vi "m100開機數統計.vi"() -> ()   [LabVIEW 2012]
uses:
  <vilib>/addons/database/Auxilliary.llb/DB Tools Cursor Type.ctl
  <vilib>/Utility/NIReport.llb/NI_report.lvclass
  <vilib>/addons/database/Connection.llb/DB Tools Open Connec (Path).vi
  <vilib>/addons/database/Connection.llb/Conn Execute.vi
  <vilib>/addons/database/Recordset.llb/Rec Fetch Recordset Data (R).vi
  <vilib>/addons/database/Recordset.llb/Rec Destroy - Connection.vi
  <vilib>/addons/database/Recordset.llb/Rec Fetch Integer Data (R).vi
  <vilib>/Utility/NIReport.llb/Append Text Table to Report (wrap).vi
  <vilib>/addons/database/_DB Variant To Data/Database Variant To Data.xnode
  <vilib>/addons/database/NI_Database_API.lvlib
  <vilib>/Utility/NIReport.llb/Excel/NI_Excel.lvclass
  <vilib>/addons/_office/NI_ReportGenerationToolkit.lvlib
panel:
  out "error out 2":errorcluster
  out "array":string[](array[string])
  out "data 3":i32
  out "data 2":string
  out "data":string
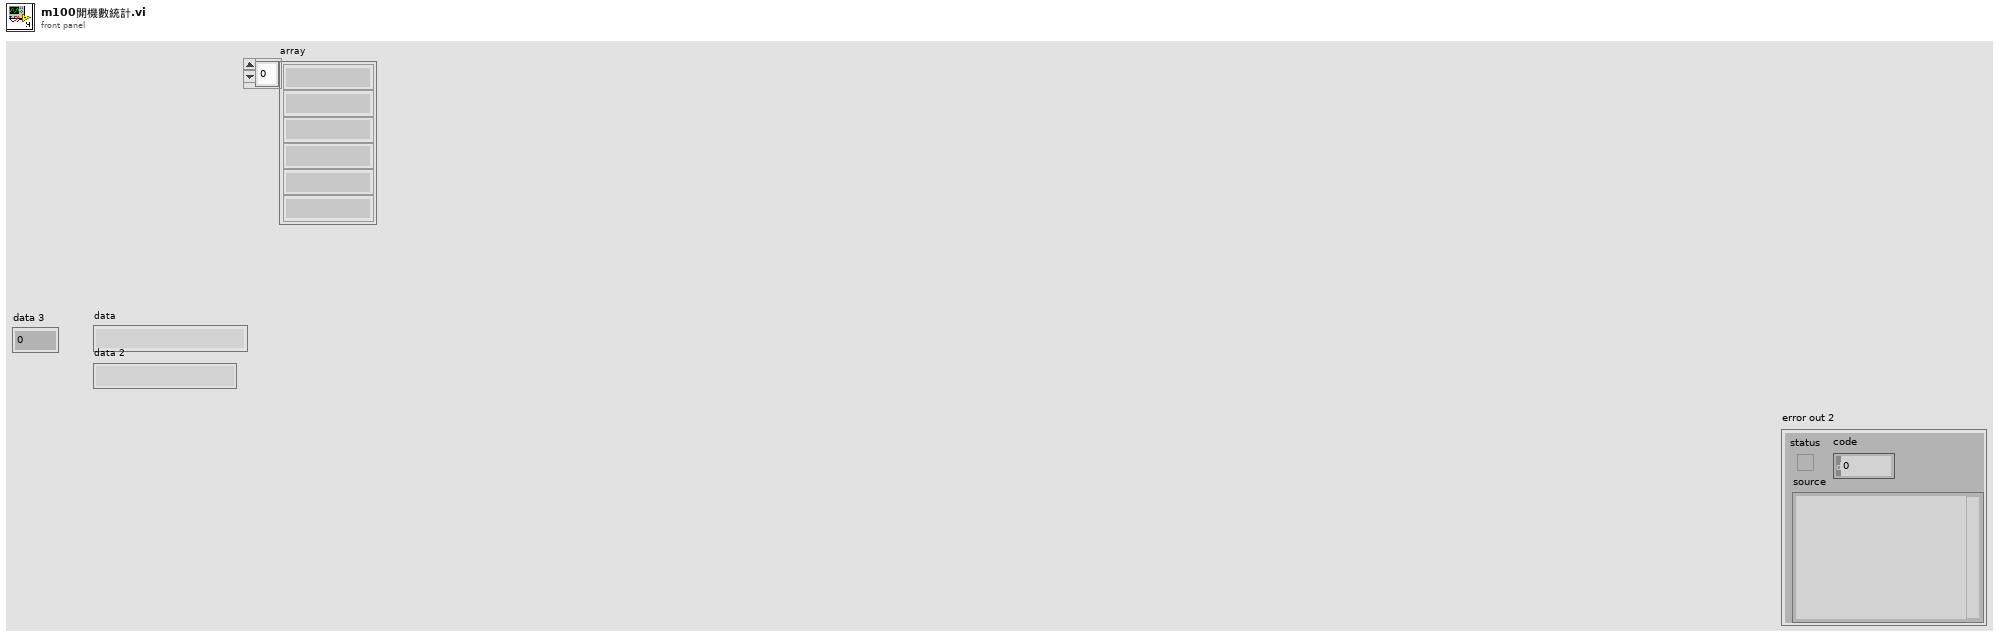
[diagram p1: front panel]
types:
  T1 = typedef "NI_Database_API.lvlib/DB Tools Cursor Type.ctl" = enum16{"forward-only", "keyset", "dynamic", "static"}
  T2 = typedef "NI_Database_API.lvlib/Conn ObjectReference.ctl" = refnum<k1>
  T3 = typedef "NI_Database_API.lvlib/Rec ObjectReference.ctl" = refnum<k1>
  T4 = enum16{"Standard Report", "HTML", "Word", "Excel"}
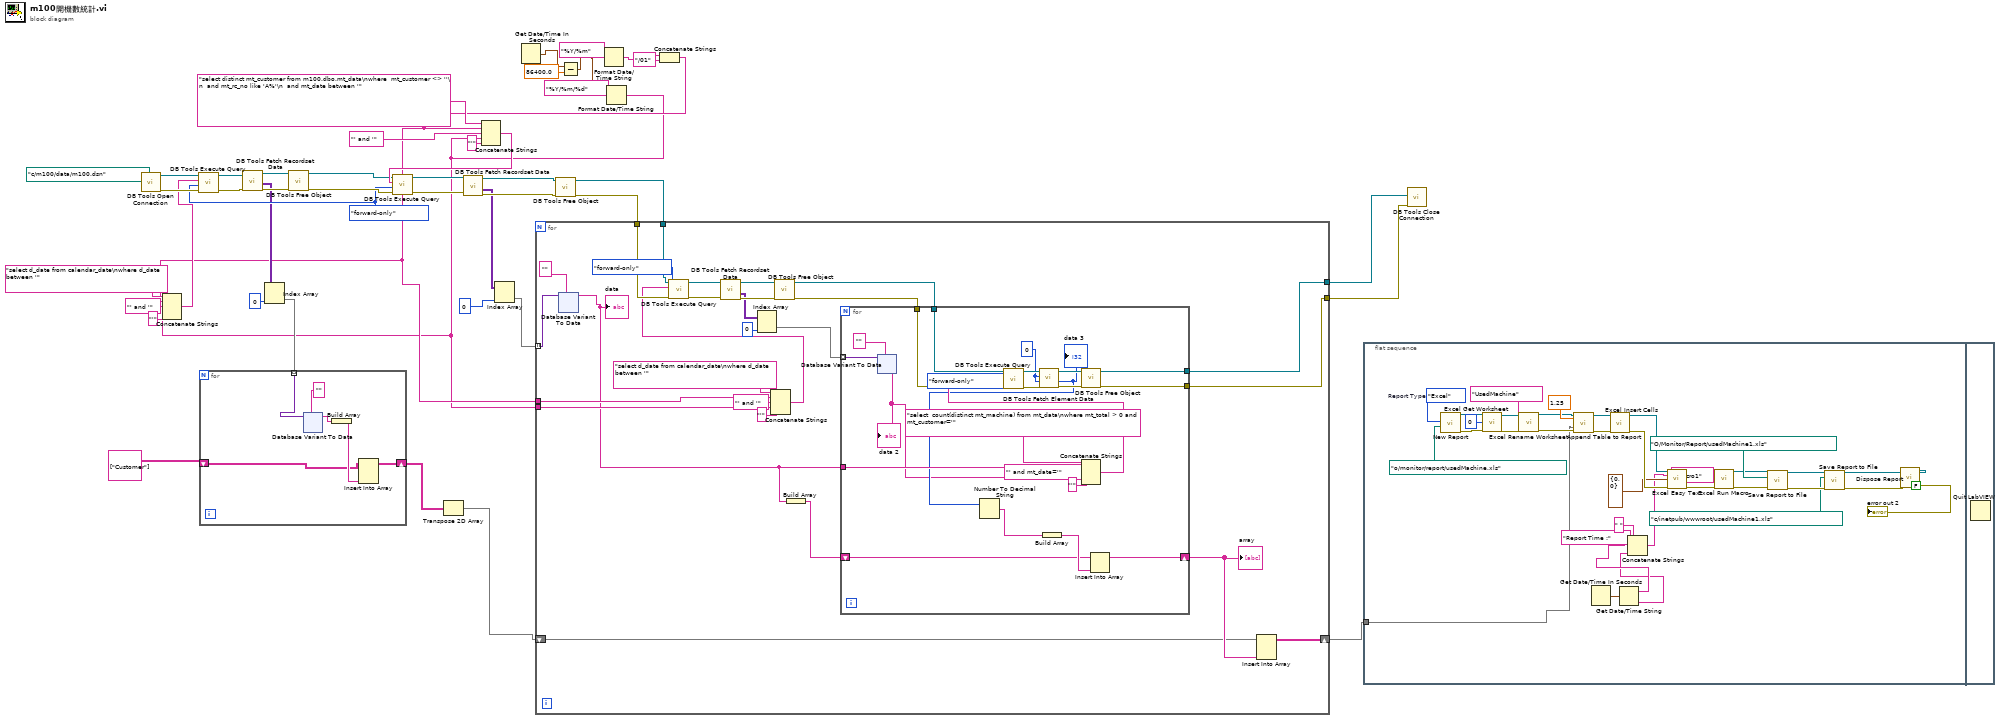
[diagram p0: block diagram]
diagram:
  w17 = DB_Tools_Cursor_Type."forward-only" ("cursor type")
  n1 = call-poly <vilib>:"DB Tools Open Connection.vi"("connection information"=path "c:/m100/data/m100.dsn") -> ("error out"=w25:errorcluster, "connection reference"=w29:T2)  [unwired: 7 in]
  n2 = Get Date/Time In Seconds() -> (seconds since 1Jan1904=w9:timestamp)
  n3 = Subtract(x=w9, y=86400.0) -> (x-y=w4:timestamp)
  n4 = Format Date/Time String(time format string (%c)="%Y/%m", seconds (now)=w4) -> (date/time string=w7:string)  [unwired: 1 in]
  n5 = Format Date/Time String(time format string (%c)="%Y/%m/%d", seconds (now)=w4) -> (date/time string=w2:string)  [unwired: 1 in]
  n6 = Concatenate Strings(w7, "/01" ("string")) -> (w3:string)
  n7 = Concatenate Strings("select d_date from calendar_date\nwhere d_date between '", w3, "' and '" ("string"), w2, "'" ("string")) -> (w18:string)
  n8 = call-poly <vilib>:"DB Tools Execute Query.vi"("error in (no error)"=w25, "cursor type"=w17, "SQL query"=w18, "connection reference"=w29) -> ("error out"=w24:errorcluster, "recordset reference"=w28:T3)  [unwired: 4 in]
  n9 = call-poly <vilib>:"DB Tools Fetch Recordset Data.vi"("error in (no error)"=w24, "recordset reference"=w28) -> ("error out"=w23:errorcluster, "recordset data"=w16:variant[][], "recordset reference out"=w27:T3)  [unwired: 3 in]
  n10 = Index Array(array=w16, index (col)=0 ("disabled index (col)")) -> (element=w15:variant[])  [unwired: 1 in]
  n11 = for {
    tunnel: w15 -> [w51] mode=indexing
    shift-right: [w47] -> w12
    shift-left: string[][] [["Customer"]] ("array") -> [w46]
    n12 = xnode "Database Variant To Data"("database variant"=w51, "type"="") -> ("data"=w49:string)  [unwired: 1 in, 1 out]
    n13 = Build Array(w49) -> (w48:string[])
    n14 = Insert Into Array(array=w46, new element=w48) -> (w47:string[][])  [unwired: 2 in]
  }
  n15 = call-poly <vilib>:"DB Tools Free Object.vi"("error in (no error)"=w23, "recordset reference"=w27) -> ("error out"=w22:errorcluster, "connection reference"=w26:T2)  [unwired: 8 in]
  n16 = Transpose 2D Array(2D array=w12) -> (transposed array=w11:string[][])
  n17 = Concatenate Strings("select distinct mt_customer from m100.dbo.mt_data\nwhere  mt_customer <> ''\n  and mt_rc_no like 'A%'\n  and mt_date between '", w3, "' and '" ("string"), w2, "'" ("string")) -> (w35:string)
  n18 = call-poly <vilib>:"DB Tools Execute Query.vi"("error in (no error)"=w22, "cursor type"=w17, "SQL query"=w35, "connection reference"=w26) -> ("error out"=w43:errorcluster, "recordset reference"=w45:T3)  [unwired: 4 in]
  n19 = call-poly <vilib>:"DB Tools Fetch Recordset Data.vi"("error in (no error)"=w43, "recordset reference"=w45) -> ("error out"=w42:errorcluster, "recordset data"=w40:variant[][], "recordset reference out"=w44:T3)  [unwired: 3 in]
  n20 = Index Array(array=w40, index (col)=0 ("disabled index (col)")) -> (element=w34:variant[])  [unwired: 1 in]
  n21 = call-poly <vilib>:"DB Tools Free Object.vi"("error in (no error)"=w42, "recordset reference"=w44) -> ("error out"=w32:errorcluster, "connection reference"=w33:T2)  [unwired: 8 in]
  n22 = for {
    tunnel: w34 -> [w109] mode=indexing
    tunnel: w33 -> [w104]
    tunnel: w32 -> [w103]
    tunnel: [w90] -> w30
    tunnel: [w89] -> w31
    tunnel: w3 -> [w101]
    tunnel: w2 -> [w99]
    shift-right: [w85] -> w1
    shift-left: w11 -> [w84]
    n23 = xnode "Database Variant To Data"("database variant"=w109, "type"="") -> ("data"=w88:string)  [unwired: 1 in, 1 out]
    "data" <- w88
    n24 = Concatenate Strings("select d_date from calendar_date\nwhere d_date between '", w101, "' and '" ("string"), w99, "'" ("string")) -> (w98:string)
    n25 = call-poly <vilib>:"DB Tools Execute Query.vi"("error in (no error)"=w103, "cursor type"=DB_Tools_Cursor_Type."forward-only", "SQL query"=w98, "connection reference"=w104) -> ("error out"=w106:errorcluster, "recordset reference"=w108:T3)  [unwired: 4 in]
    n26 = call-poly <vilib>:"DB Tools Fetch Recordset Data.vi"("error in (no error)"=w106, "recordset reference"=w108) -> ("error out"=w105:errorcluster, "recordset data"=w96:variant[][], "recordset reference out"=w107:T3)  [unwired: 3 in]
    n27 = Index Array(array=w96, index (col)=0 ("disabled index (col)")) -> (element=w95:variant[])  [unwired: 1 in]
    n28 = call-poly <vilib>:"DB Tools Free Object.vi"("error in (no error)"=w105, "recordset reference"=w107) -> ("error out"=w91:errorcluster, "connection reference"=w92:T2)  [unwired: 8 in]
    n29 = Build Array(w88) -> (w87:string[])
    n30 = for {
      tunnel: w95 -> [w133] mode=indexing
      tunnel: w92 -> [w127]
      tunnel: w91 -> [w126]
      tunnel: [w125] -> w90
      tunnel: [w124] -> w89
      tunnel: w88 -> [w117]
      shift-right: [w114] -> w86
      shift-left: w87 -> [w113]
      w118 = 0
      n31 = xnode "Database Variant To Data"("database variant"=w133, "type"="") -> ("data"=w111:string)  [unwired: 1 in, 1 out]
      "data 2" <- w111
      n32 = Concatenate Strings("select  count(distinct mt_machine) from mt_data\nwhere mt_total > 0 and mt_customer='", w117, "' and mt_date='" ("string"), w111, "'" ("string")) -> (w120:string)
      n33 = call-poly <vilib>:"DB Tools Execute Query.vi"("error in (no error)"=w126, "cursor type"=DB_Tools_Cursor_Type."forward-only", "SQL query"=w120, "connection reference"=w127) -> ("error out"=w129:errorcluster, "recordset reference"=w131:T3)  [unwired: 4 in]
      n34 = call-poly <vilib>:"DB Tools Fetch Element Data.vi"("error in (no error)"=w129, "type"=w118, "column index"=w118, "recordset reference"=w131) -> ("error out"=w128:errorcluster, "data"=w116:i32, "recordset reference out"=w130:T3)  [unwired: 3 in]
      "data 3" <- w116
      n35 = Number To Decimal String(number=w116) -> (decimal integer string=w112:string)  [unwired: 1 in]
      n36 = Build Array(w112) -> (w115:string[])
      n37 = call-poly <vilib>:"DB Tools Free Object.vi"("error in (no error)"=w128, "recordset reference"=w130) -> ("error out"=w124:errorcluster, "connection reference"=w125:T2)  [unwired: 8 in]
      n38 = Insert Into Array(array=w113, new element=w115) -> (w114:string[])  [unwired: 1 in]
    }
    "array" <- w86
    n39 = Insert Into Array(array=w84, new element=w86) -> (w85:string[][])  [unwired: 2 in]
  }
  n40 = flat-sequence {
    tunnel: w1 -> [w203]
    frame #0 {
      w233 = T4."Excel"  # Report Type
      n41 = call <vilib>:"New Report.vi"("report type"=w233, "template (empty)"=path "o:/monitor/report/usedMachine.xls" ("Report Template")) -> ("report out"=w228:refnum<class "NI_report.lvclass">, "error out"=w227:errorcluster)  [unwired: 12 in]
      n42 = call <vilib>:"Excel Get Worksheet.vi"("report in"=w228, "worksheet index (0)"=0, "error in (no error)"=w227) -> ("report out"=w225:refnum<class "NI_report.lvclass">, "error out"=w223:errorcluster)  [unwired: 11 in]
      n43 = call <vilib>:"Excel Rename Worksheet.vi"("report in"=w225, "worksheet name (\"\")"="UsedMachine" ("worksheet name (\"\")"), "error in (no error)"=w223) -> ("report out"=w224:refnum<class "NI_report.lvclass">, "error out"=w222:errorcluster)  [unwired: 11 in]
      n44 = call-poly <vilib>:"Append Table to Report.vi"("report in"=w224, "column width (1)"=1.25, "text data"=w203, "error in (no error)"=w222) -> ("report out"=w230:refnum<class "NI_report.lvclass">, "error out"=w229:errorcluster)  [unwired: 8 in, 2 out]
      n45 = Get Date/Time In Seconds() -> (seconds since 1Jan1904=w216:timestamp)
      n46 = call <vilib>:"Excel Insert Cells.vi"("report in"=w230, "error in (no error)"=w229) -> ("report out"=w220:refnum<class "NI_report.lvclass">, "error out"=w219:errorcluster)  [unwired: 12 in]
      n47 = Get Date/Time String(seconds (now)=w216) -> (date string=w215:string, time string=w213:string)  [unwired: 2 in]
      n48 = Concatenate Strings("Report Time :" ("string"), w215, " " ("string"), w213) -> (w212:string)
      n49 = call <vilib>:"Excel Easy Text.vi"("report in"=w220, "text"=w212, "start (-1, -1)"=cluster{"row":i32, "column":i32} {"row"=0, "column"=0} ("end (-1, -1)"), "error in (no error)"=w219) -> ("report out"=w202:refnum<class "NI_report.lvclass">, "error out"=w200:errorcluster)  [unwired: 7 in, 3 out]
      n50 = call <vilib>:"Excel Run Macro.vi"("report in"=w202, "macro name"="macro1", "error in (no error)"=w200) -> ("report out"=w201:refnum<class "NI_report.lvclass">, "error out"=w199:errorcluster)  [unwired: 10 in, 1 out]
      n51 = call-dynamic "Save Report to File.vi"("report in"=w201, "report file path"=path "O:/Monitor/Report/usedMachine1.xls", "error in (no error)"=w199) -> ("report out"=w208:refnum<class "NI_report.lvclass">, "error out"=w206:errorcluster)  [unwired: 11 in]
      n52 = call-dynamic "Save Report to File.vi"("report in"=w208, "report file path"=path "c:/inetpub/wwwroot/usedMachine1.xls", "error in (no error)"=w206) -> ("report out"=w207:refnum<class "NI_report.lvclass">, "error out"=w205:errorcluster)  [unwired: 11 in]
      n53 = call-dynamic "Dispose Report.vi"("report in"=w207, "save changes? (F)"=FALSE, "error in (no error)"=w205) -> ("error out"=→"error out 2":errorcluster)  [unwired: 12 in]
    }
    frame #1 {
      n54 = Quit LabVIEW() -> ()  [unwired: 1 in]
    }
  }
  n55 = call <vilib>:"DB Tools Close Connection.vi"("error in (no error)"=w31, "connection reference"=w30) -> ()  [unwired: 5 in, 1 out]
